vi "StringWizard.vi"() -> ()   [LabVIEW 2020]
uses:
  vi-prop-cmd.ctl
  <vilib>/Utility/miscctls.llb/LVRowAndColumnUnsignedTypeDef.ctl
  <vilib>/ErrorRing/Error Ring.xnode
panel:
  in  "reload":bool
  in  "Directory":path
  in  "Multicolumn Listbox":i32(listbox)
  in  "open":bool
  out "Icon":picture
  in  "Custom":bool
  in  "Description":string
  in  "Title":string
  out "VI Name":string
  in  "control strings":i32(listbox)
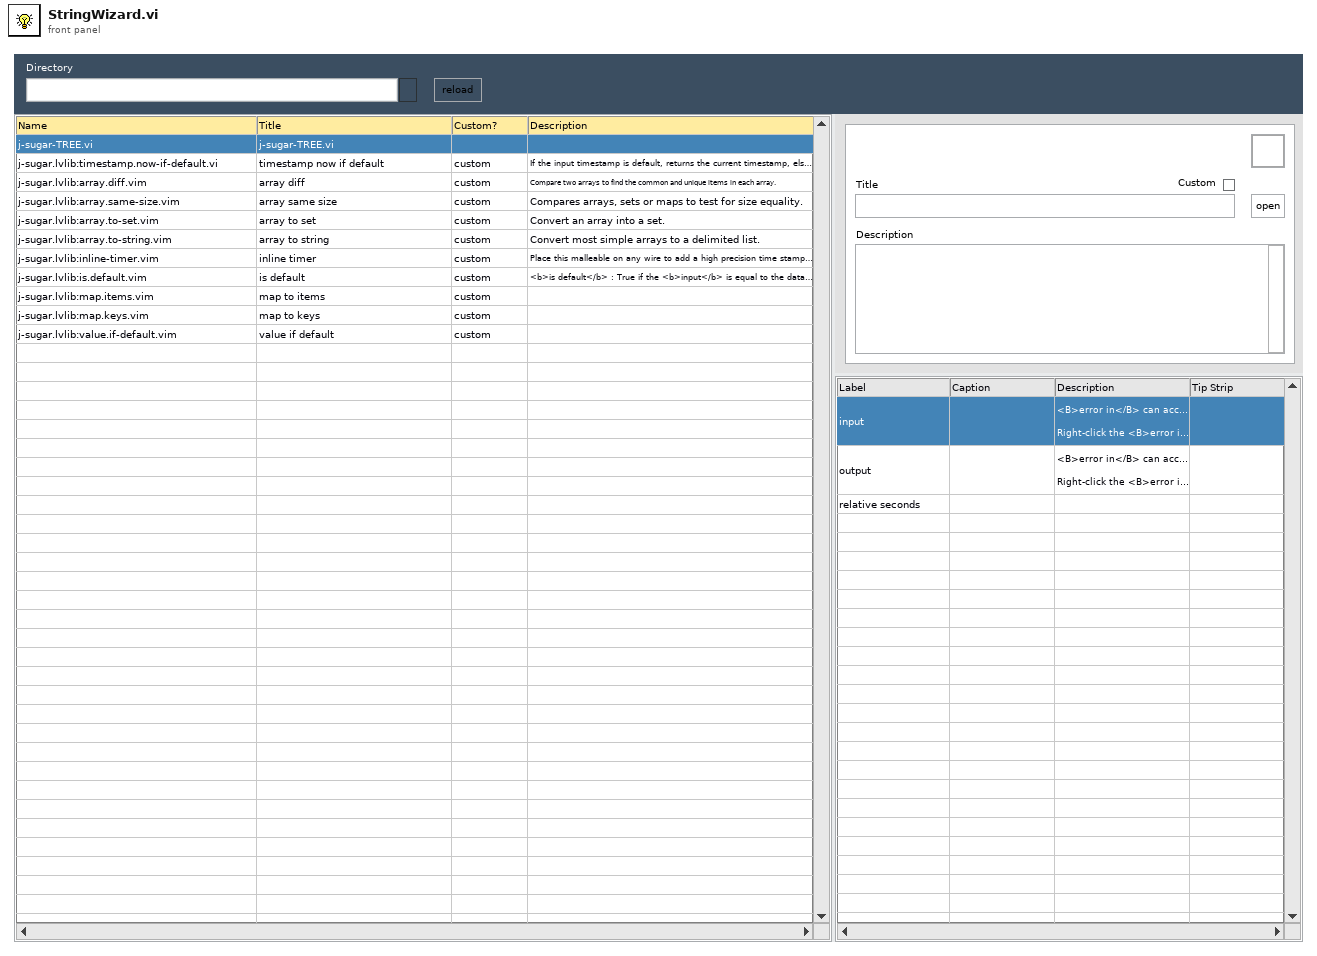
[diagram p1: front panel]
types:
  T1 = enum32{"Invalid", "Standard", "Closed", "Hidden", "Minimized", "Maximized"}
  T2 = enum32{"invalid app kind", "Development System", "Run Time System", "Student Edition", "Embedded LabVIEW", "Evaluation", "Custom"}
  T3 = typedef "LVRowAndColumnUnsignedTypeDef.ctl" = cluster{"Row":u32, "Column":u32}
  T4 = typedef "vi-prop-cmd.ctl" = cluster{"vi path":path, "property":string, "val":variant}
  T5 = cluster{"Core":cluster{"Current VI Reference":refnum<vi>, "Close Panel on Exit?":bool}, "mclb":refnum<vi>, "payload":T4, "Directory":path, "selected VI":path}
  T6 = typedef "LVRowAndColumnTypeDef.ctl" = cluster{"Row":i32, "Column":i32}
  T7 = cluster{"Current VI Reference":refnum<vi>, "Close Panel on Exit?":bool}
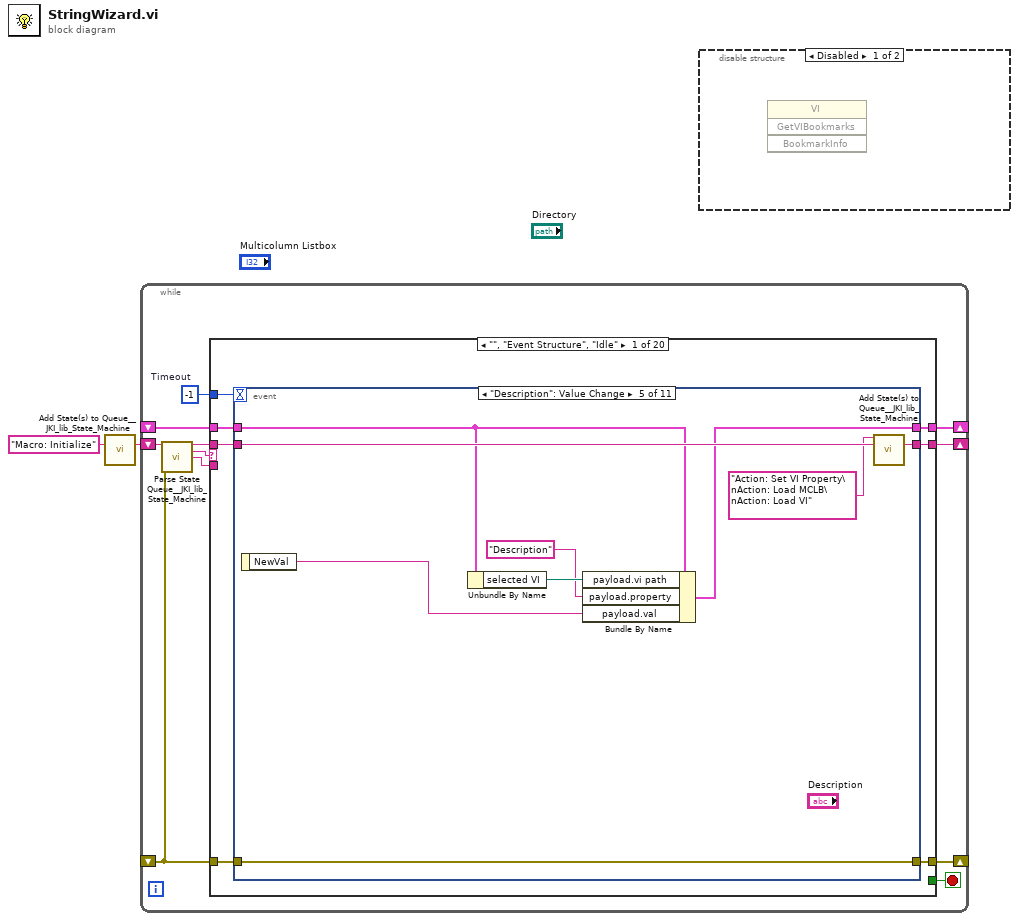
[diagram p0: block diagram]
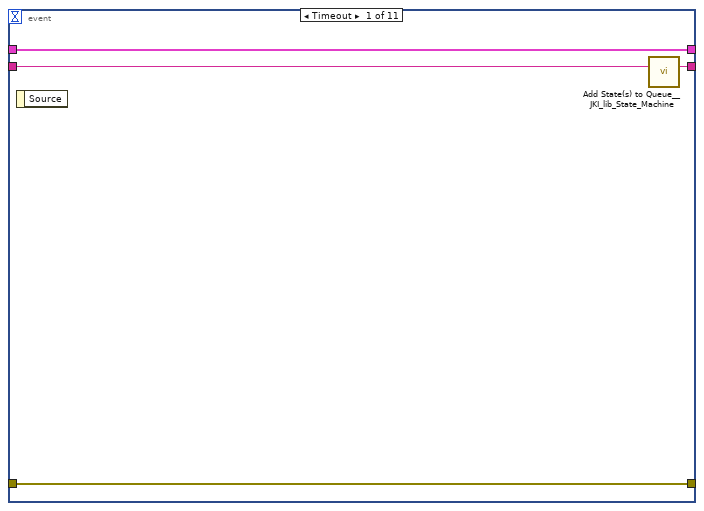
[diagram p3: hidden frame]
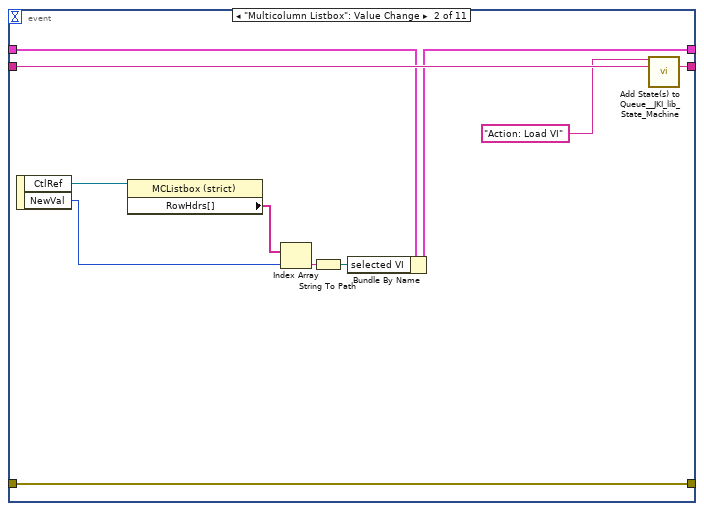
[diagram p4: hidden frame]
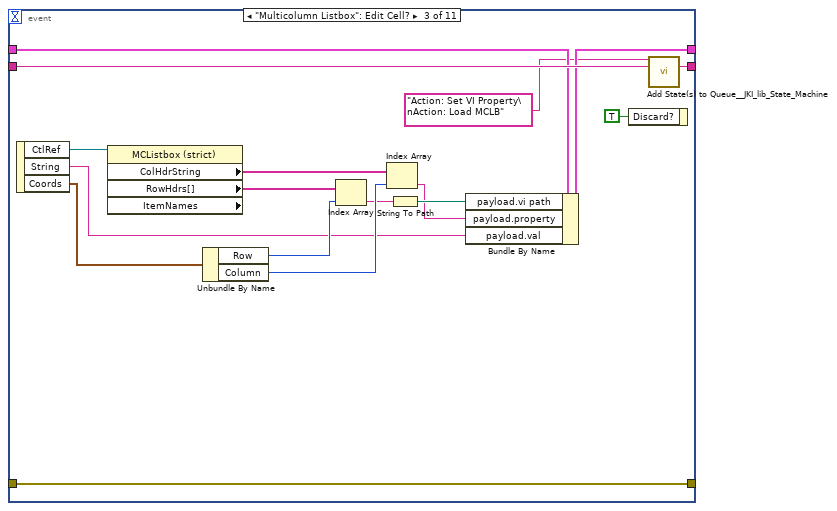
[diagram p5: hidden frame]
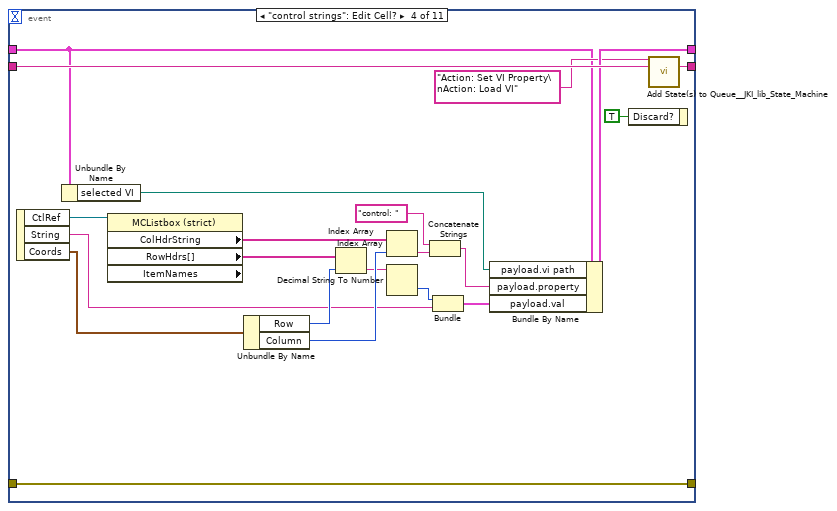
[diagram p6: hidden frame]
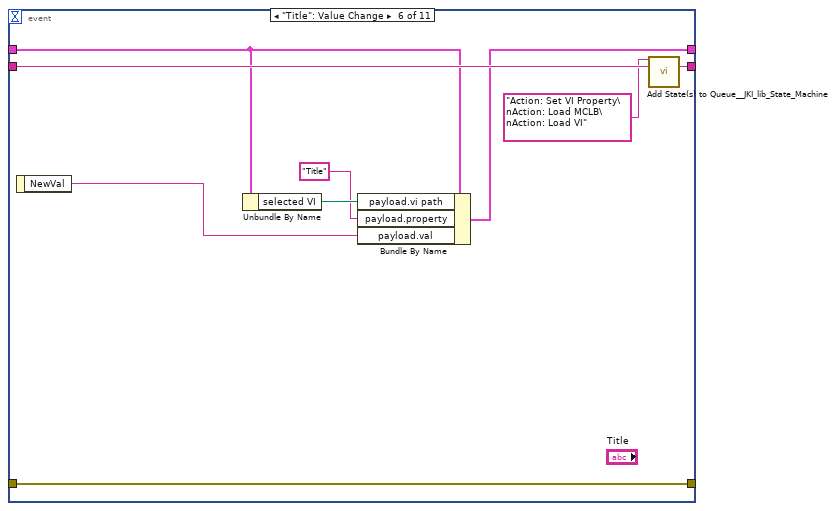
[diagram p7: hidden frame]
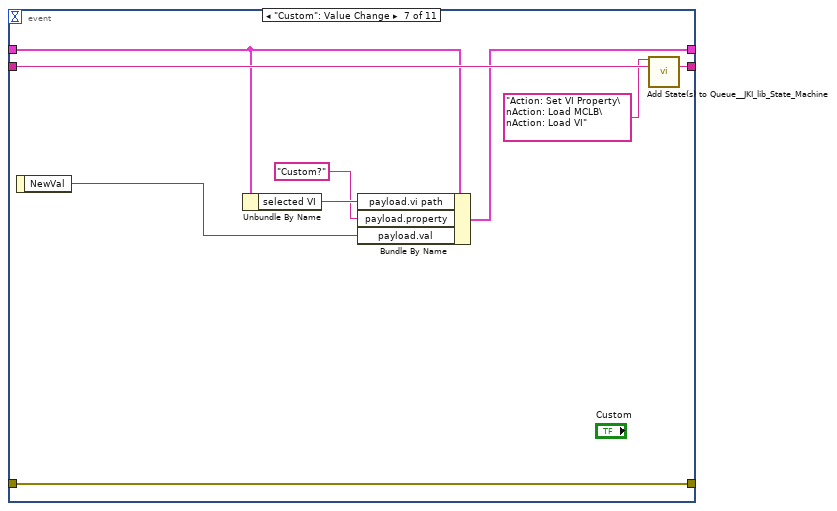
[diagram p8: hidden frame]
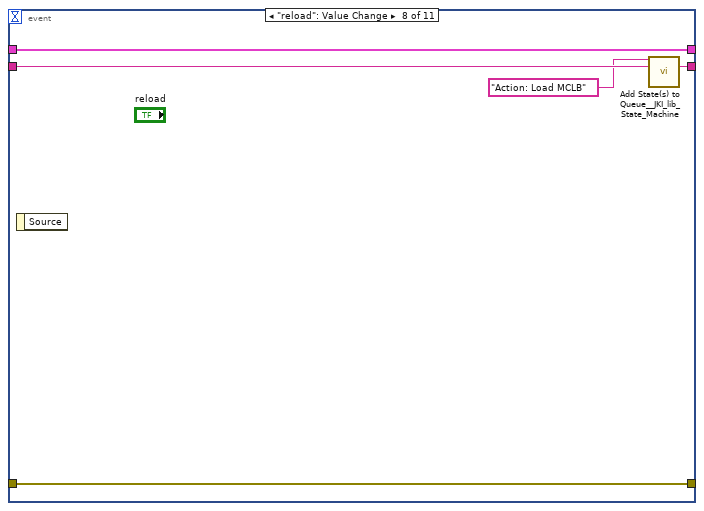
[diagram p9: hidden frame]
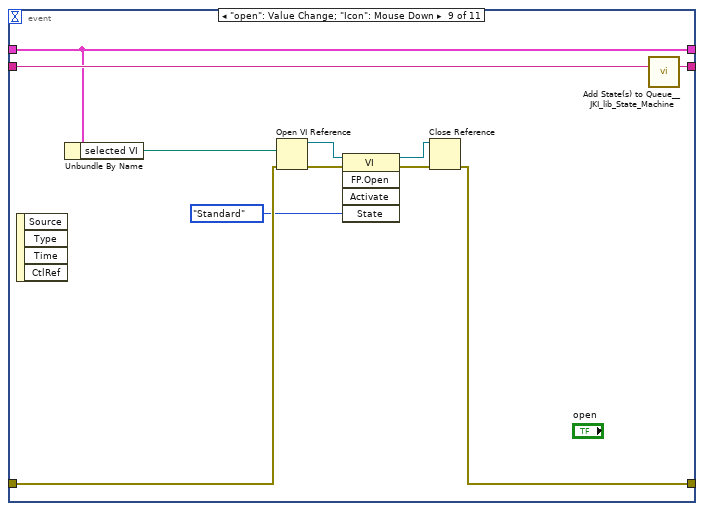
[diagram p10: hidden frame]
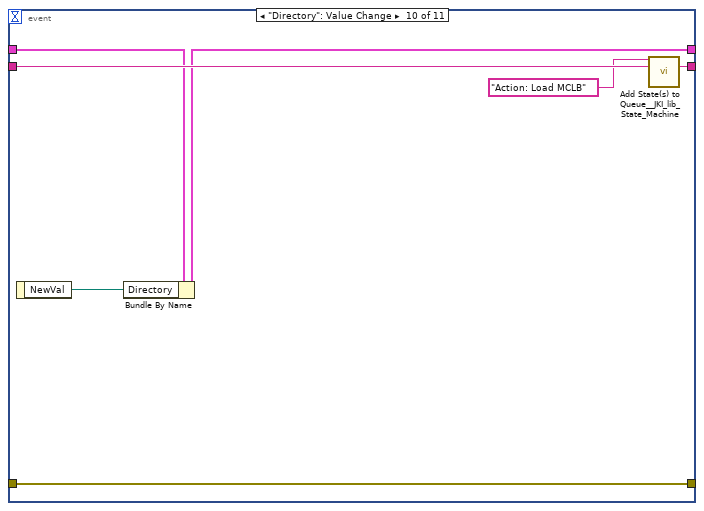
[diagram p11: hidden frame]
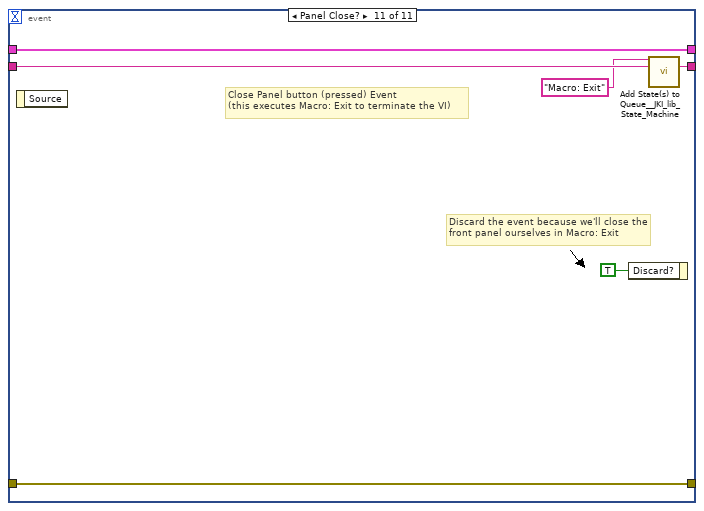
[diagram p12: hidden frame]
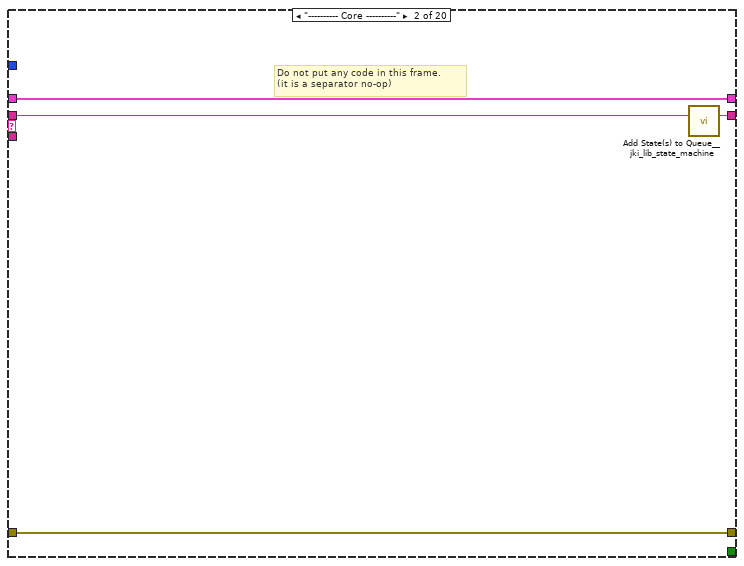
[diagram p13: hidden frame]
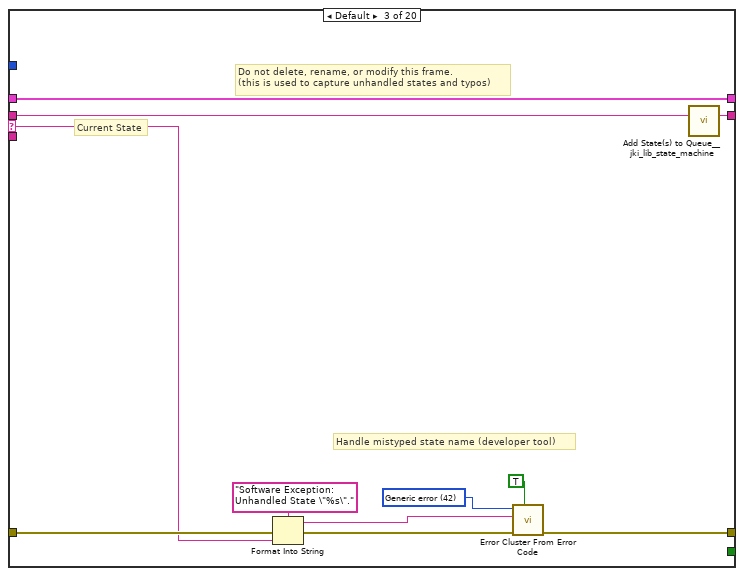
[diagram p14: hidden frame]
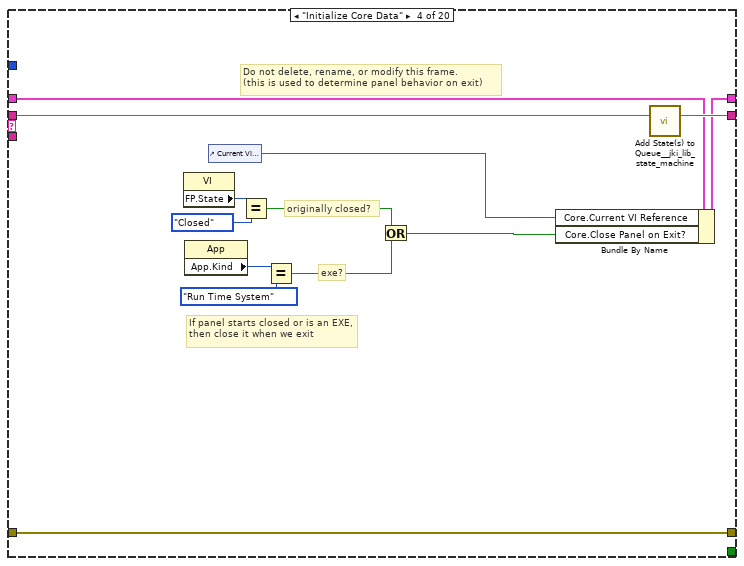
[diagram p15: hidden frame]
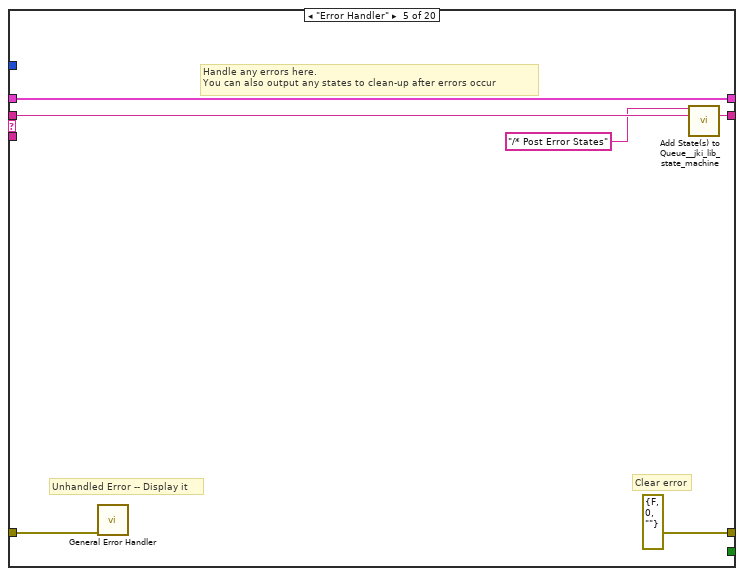
[diagram p16: hidden frame]
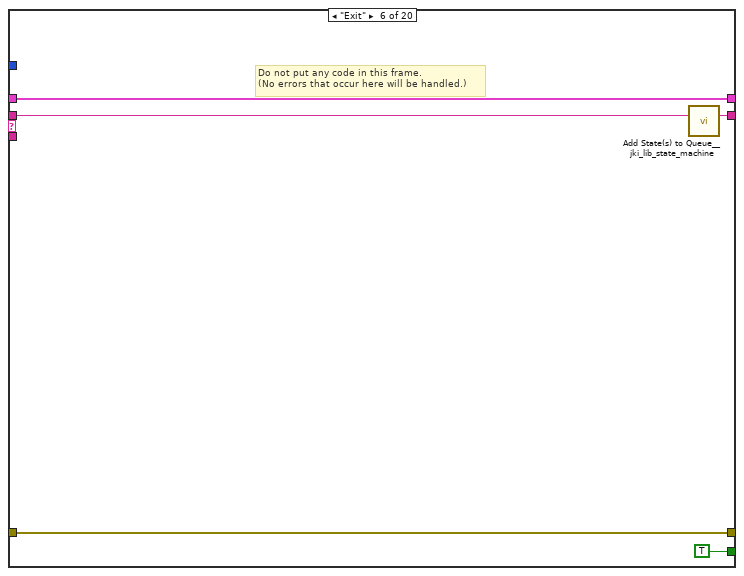
[diagram p17: hidden frame]
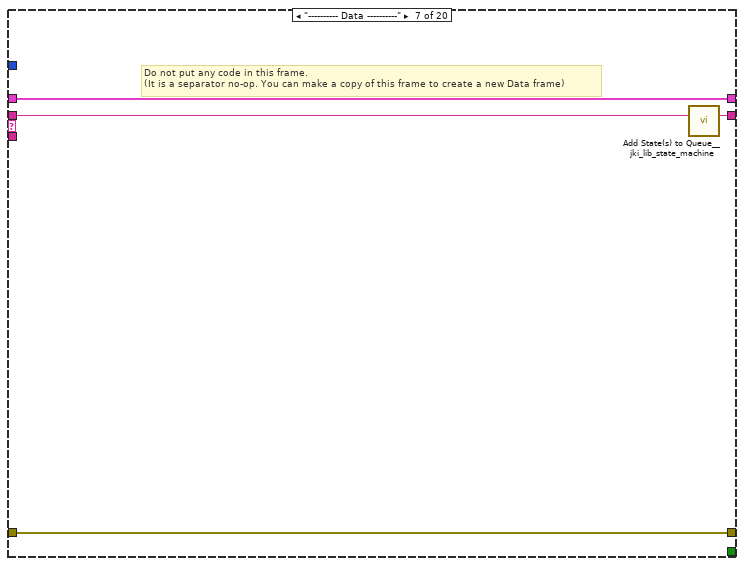
[diagram p18: hidden frame]
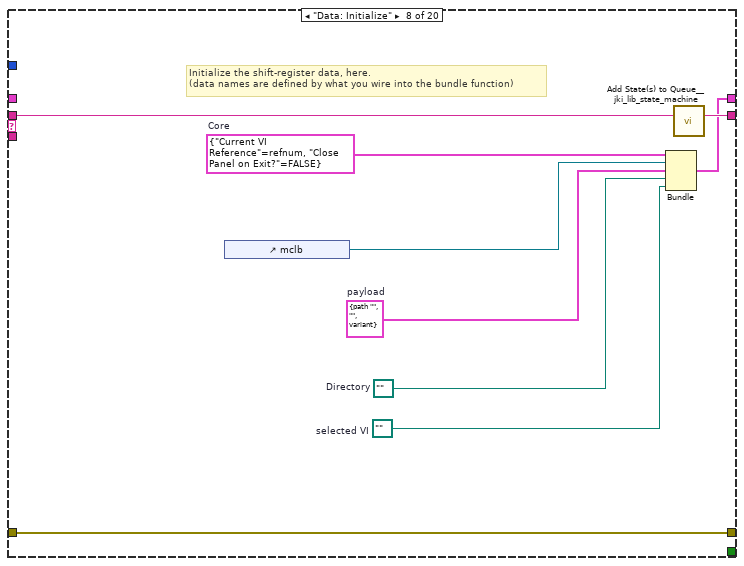
[diagram p19: hidden frame]
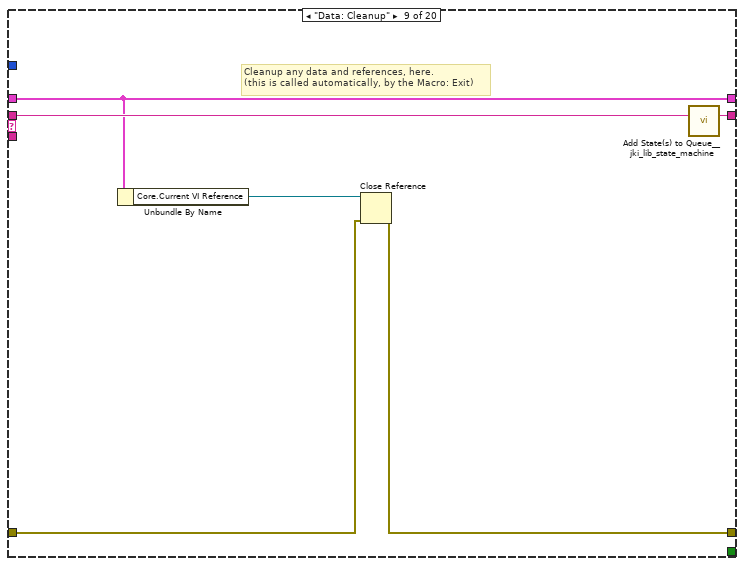
[diagram p20: hidden frame]
diagram:
  n1 = call <vilib>:"Add State(s) to Queue__JKI_lib_State_Machine.vi"("State(s) in (\"\")"="Macro: Initialize") -> ("States Out"=w2:string)  [unwired: 14 in]
  n2 = while {
    shift-right: [w6] -> _
    shift-left: _ -> [w5]
    shift-right: [w9] -> _
    shift-left: _ -> [w3]
    shift-right: [w8] -> _
    shift-left: w2 -> [w10]
    stop <- w7 stop-if-true
    w4 = -1  # Timeout
    n3 = call <vilib>:"Parse State Queue__JKI_lib_State_Machine.vi"("State Queue"=w10, "Error In (no error)"=w3) -> ("Remaining States"=w12:string, "Current State"=w13:string, "Arguments"=w11:string)  [unwired: 11 in]
    n4 = case shown="\"\", \"Event Structure\", \"Idle\"" w13 {
      selector: w13 -> [_ _ w134 _ _ _ _ _ _ _ _ _ _ _ _ _ _ _ _ _]
      tunnel: w12 -> [w20 w133 w138 w157 w163 w168 w172 w181 w187 w191 w203 w211 w222 w291 w296 w306 w310 w333 w350 w420]
      tunnel: w11 -> [_ _ _ _ _ _ _ _ _ _ _ w206 w216 _ _ _ _ _ _ _]
      tunnel: w5 -> [w18 w130 w136 w150 w160 w166 w169 _ w183 w188 w201 w209 w218 w288 w293 w303 w307 w331 w337 w413]
      tunnel: [w17 w131 w140 w154 errorcluster {"status"=FALSE, "code"=0, "source"=""} ("error out") w165 w170 w175 w184 w189 w200 w207 w219 w289 w294 w304 w308 w323 w335 w410] -> w9
      tunnel: w3 -> [w16 w131 w139 w154 w159 w165 w170 w175 w182 w189 w200 w208 w220 w289 w294 w304 w308 w330 w334 w411]
      tunnel: [w19 w132 w137 w156 w162 w167 w171 w180 w186 w190 w202 w210 w221 w290 w295 w305 w309 w332 w349 w419] -> w8
      tunnel: [_ _ _ _ _ TRUE _ _ _ _ _ _ _ _ _ _ _ _ _ _] -> w7
      tunnel: [w15 w130 w136 w155 w160 w166 w169 w179 w183 w188 w201 w209 w218 w288 w293 w303 w307 w331 w338 w413] -> w6
      tunnel: w4 -> [w14 _ _ _ _ _ _ _ _ _ _ _ _ _ _ _ _ _ _ _]
      frame "", "Event Structure", "Idle" {
        n5 = event shown="[4] \"Description\": Value Change" {
          selector: _ -> [_ _ _ _ _ _ _ _ _ _ _]
          dyn-events: _ -> [_ _ _ _ _ _ _ _ _ _ _]
          timeout: w14 -> [_ _ _ _ _ _ _ _ _ _ _]
          tunnel: w20 -> [w24 w35 w52 w73 w82 w91 w100 w105 w116 w123 w129]
          tunnel: [w23 w34 w51 w72 w81 w90 w99 w104 w115 w122 w128] -> w19
          tunnel: w18 -> [w21 w32 w44 w61 w77 w86 w95 w102 w114 w117 w126]
          tunnel: [w22 w33 w50 w71 w80 w89 w98 w103 w109 w121 w127] -> w17
          tunnel: w16 -> [w22 w33 w50 w71 w80 w89 w98 w103 w108 w121 w127]
          tunnel: [w21 w26 w45 w66 w79 w88 w97 w102 w114 w118 w126] -> w15
          event Timeout {
            n6 = event-data() -> ()  [unwired: 1 in, 1 out]
            n7 = call <vilib>:"Add State(s) to Queue__JKI_lib_State_Machine.vi"("State(s) in (\"\")"=w24) -> ("States Out"=w23:string)  [unwired: 14 in]
          }
          event "Multicolumn Listbox": Value Change {
            n8 = event-data() -> ("CtlRef"=w31:refnum<vi>, "NewVal"=w29:i32)  [unwired: 1 in]
            n9 = property on="Property Node" class="MCListbox (strict)"(reference=w31) -> ("RowHdrs[]"=w30:string[])  [unwired: 1 in, 2 out]
            n10 = Index Array(array=w30, index=w29) -> (element=w28:string)
            n11 = String To Path(string=w28) -> (path=w25:path)
            n12 = Bundle By Name(cluster=w32, "selected VI"=w25) -> (w26:T5)
            n13 = call <vilib>:"Add State(s) to Queue__JKI_lib_State_Machine.vi"("State(s) in Front (\"\")"="Action: Load VI", "State(s) in (\"\")"=w35) -> ("States Out"=w34:string)  [unwired: 13 in]
          }
          event "Multicolumn Listbox": Edit Cell? {
            n14 = event-data() -> ("CtlRef"=w47:refnum<vi>, "String"=w38:string, "Coords"=w36:T6)  [unwired: 1 in]
            n15 = property on="Property Node" class="MCListbox (strict)" props=["ColHdrString", "RowHdrs[]", "ItemNames"](reference=w47) -> ("ColHdrString"=w49:string[], "RowHdrs[]"=w48:string[])  [unwired: 1 in, 3 out]
            n16 = Unbundle By Name(w36) -> ("Row"=w43:i32, "Column"=w42:i32)
            n17 = Index Array(array=w48, index=w43) -> (element=w41:string)
            n18 = Index Array(array=w49, index=w42) -> (element=w39:string)
            n19 = String To Path(string=w41) -> (path=w40:path)
            n20 = Bundle By Name(cluster=w44, "payload.vi path"=w40, "payload.property"=w39, "payload.val"=w38) -> (w45:T5)
            n21 = event-data("Discard?"=TRUE) -> ()  [unwired: 1 in, 1 out]
            n22 = call <vilib>:"Add State(s) to Queue__JKI_lib_State_Machine.vi"("State(s) in Front (\"\")"="Action: Set VI Property\nAction: Load MCLB", "State(s) in (\"\")"=w52) -> ("States Out"=w51:string)  [unwired: 13 in]
          }
          event "control strings": Edit Cell? {
            n23 = event-data() -> ("CtlRef"=w68:refnum<vi>, "String"=w56:string, "Coords"=w62:T6)  [unwired: 1 in]
            n24 = Unbundle By Name(w61) -> ("selected VI"=w60:path)
            n25 = property on="Property Node" class="MCListbox (strict)" props=["ColHdrString", "RowHdrs[]", "ItemNames"](reference=w68) -> ("ColHdrString"=w70:string[], "RowHdrs[]"=w69:string[])  [unwired: 1 in, 3 out]
            n26 = Unbundle By Name(w62) -> ("Row"=w65:i32, "Column"=w64:i32)
            n27 = Index Array(array=w69, index=w65) -> (element=w54:string)
            n28 = Index Array(array=w70, index=w64) -> (element=w58:string)
            n29 = Decimal String To Number(string=w54) -> (number=w53:i32)  [unwired: 2 in, 1 out]
            n30 = Concatenate Strings("control: ", w58) -> (w57:string)
            n31 = Bundle(w53, "String"=w56) -> (w55:cluster{i32, "String":string})  [unwired: 1 in]
            n32 = Bundle By Name(cluster=w61, "payload.vi path"=w60, "payload.property"=w57, "payload.val"=w55) -> (w66:T5)
            n33 = event-data("Discard?"=TRUE) -> ()  [unwired: 1 in, 1 out]
            n34 = call <vilib>:"Add State(s) to Queue__JKI_lib_State_Machine.vi"("State(s) in Front (\"\")"="Action: Set VI Property\nAction: Load VI", "State(s) in (\"\")"=w73) -> ("States Out"=w72:string)  [unwired: 13 in]
          }
          event "Description": Value Change {
            n35 = event-data() -> ("NewVal"=w76:string)  [unwired: 1 in]
            n36 = Unbundle By Name(w77) -> ("selected VI"=w75:path)
            n37 = Bundle By Name(cluster=w77, "payload.vi path"=w75, "payload.property"="Description", "payload.val"=w76) -> (w79:T5)
            n38 = call <vilib>:"Add State(s) to Queue__JKI_lib_State_Machine.vi"("State(s) in Front (\"\")"="Action: Set VI Property\nAction: Load MCLB\nAction: Load VI", "State(s) in (\"\")"=w82) -> ("States Out"=w81:string)  [unwired: 13 in]
          }
          event "Title": Value Change {
            n39 = event-data() -> ("NewVal"=w85:string)  [unwired: 1 in]
            n40 = Unbundle By Name(w86) -> ("selected VI"=w84:path)
            n41 = Bundle By Name(cluster=w86, "payload.vi path"=w84, "payload.property"="Title", "payload.val"=w85) -> (w88:T5)
            n42 = call <vilib>:"Add State(s) to Queue__JKI_lib_State_Machine.vi"("State(s) in Front (\"\")"="Action: Set VI Property\nAction: Load MCLB\nAction: Load VI", "State(s) in (\"\")"=w91) -> ("States Out"=w90:string)  [unwired: 13 in]
          }
          event "Custom": Value Change {
            n43 = event-data() -> ("NewVal"=w94:bool)  [unwired: 1 in]
            n44 = Unbundle By Name(w95) -> ("selected VI"=w93:path)
            n45 = Bundle By Name(cluster=w95, "payload.vi path"=w93, "payload.property"="Custom?", "payload.val"=w94) -> (w97:T5)
            n46 = call <vilib>:"Add State(s) to Queue__JKI_lib_State_Machine.vi"("State(s) in Front (\"\")"="Action: Set VI Property\nAction: Load MCLB\nAction: Load VI", "State(s) in (\"\")"=w100) -> ("States Out"=w99:string)  [unwired: 13 in]
          }
          event "reload": Value Change {
            n47 = event-data() -> ()  [unwired: 1 in, 1 out]
            n48 = call <vilib>:"Add State(s) to Queue__JKI_lib_State_Machine.vi"("State(s) in Front (\"\")"="Action: Load MCLB", "State(s) in (\"\")"=w105) -> ("States Out"=w104:string)  [unwired: 13 in]
          }
          event "open": Value Change; "Icon": Mouse Down {
            n49 = event-data() -> ()  [unwired: 1 in, 4 out]
            n50 = Unbundle By Name(w114) -> ("selected VI"=w113:path)
            n51 = Open VI Reference(vi path=w113, error in (no error)=w108) -> (vi reference=w106:refnum<vi>, error out=w112:errorcluster)  [unwired: 4 in]
            n52 = invoke class="VI" method="FP.Open"(reference=w106, error in=w112, "State"=T1."Standard") -> (reference out=w110:refnum<vi>, error out=w111:errorcluster)  [unwired: 2 in, 3 out]
            n53 = Close Reference(reference=w110, error in (no error)=w111) -> (error out=w109:errorcluster)
            n54 = call <vilib>:"Add State(s) to Queue__JKI_lib_State_Machine.vi"("State(s) in (\"\")"=w116) -> ("States Out"=w115:string)  [unwired: 14 in]
          }
          event "Directory": Value Change {
            n55 = event-data() -> ("NewVal"=w119:path)  [unwired: 1 in]
            n56 = Bundle By Name(cluster=w117, "Directory"=w119) -> (w118:T5)
            n57 = call <vilib>:"Add State(s) to Queue__JKI_lib_State_Machine.vi"("State(s) in Front (\"\")"="Action: Load MCLB", "State(s) in (\"\")"=w123) -> ("States Out"=w122:string)  [unwired: 13 in]
          }
          event Panel Close? {
            # "Discard the event because we'll close the front panel ourselves in Macro: Exit"
            # "Close Panel button (pressed) Event\n(this executes Macro: Exit to terminate the VI)"
            n58 = event-data() -> ()  [unwired: 1 in, 1 out]
            n59 = event-data("Discard?"=TRUE) -> ()  [unwired: 1 in, 1 out]
            n60 = call <vilib>:"Add State(s) to Queue__JKI_lib_State_Machine.vi"("State(s) in Front (\"\")"="Macro: Exit", "State(s) in (\"\")"=w129) -> ("States Out"=w128:string)  [unwired: 13 in]
          }
        }
      }
      frame "---------- Core ----------" {
        # "Do not put any code in this frame.\n(it is a separator no-op)"
        n61 = call <vilib>:"Add State(s) to Queue__jki_lib_state_machine.vi"("State(s) in (\"\")"=w133) -> ("States Out"=w132:string)  [unwired: 14 in]
      }
      frame Default {
        w143 = 42 items=["No error", "Argument error", "Memory is full", "Out of zone", "End of file", "File already open", "Generic file I/O error", "File not found", "File permission error", "Disk is full", "Duplicate path", "Too many files open", "System feature not enabled", "Resource file not found", "Cannot add resource", "Resource not found", "Image not found", "Image memory error", "Pen does not exist", "Config type invalid", "Config token not found", "Config parse error", "Config memory error", "Bad external code format", "Bad external code offset", "External code not present", "Null window", "Destroy window error", "Null menu", "Print aborted", "Bad print record", "Print driver error", "Windows error during printing", "Memory error during printing", "Print dialog error", "Generic print error", "Invalid device refnum", "Device not found", "Device parameter error", "Device unit error", "Cannot open device", "Device call aborted", "Generic error", "Cancelled by user", "Object ID too low", "Object ID too high", "Object not in heap", "Unknown heap", "Unknown object (invalid DefProc)", "Unknown object (DefProc not in table)", "Message out of range", "Invalid (null) method", "Unknown message", "Manager call not supported", "Bad address", "Network operation in progress", "Network operation timed out", "Connection is busy", "Network attribute not supported", "Network error", "Address in use", "System out of memory", "Connection aborted", "Connection refused", "Not connected", "Already connected", "Connection closed", "Initialization error (interapplication manager)", "Bad occurrence", "Wait on unbound occurrence handler", "Occurrence queue overflow", "Datalog type conflict", "Unused", "Unrecognized type (interapplication manager)", "Memory corrupt", "Failed to make temporary DLL", "Old CIN version", "Drag socket not found", "Failed to load drop-object", "Failed to register OLE object", "Failed to release OLE object", "Format specifier type mismatch", "Unknown format specifier", "Too few format specifiers", "Too many format specifiers", "Scan failed", "Newer CIN version", "Error converting to variant", "Runtime menu error", "Password tampered", "Variant attribute not found", "Incompatible variant data type", "Event data is not available", "Event Store is not present", "Occurrence is not found", "Event Queue is not created", "Event info is not available", "Refnum passed is NULL", "Error retrieving Class GUID", "Error retrieving CoClass GUID", "Error retrieving TypeLib GUID.", "Bad built application magic bytes.", "Specific driver is different from the specific driver associated with the Logical Name.", "There is no session opened to the class driver.", "Max Error", "MAX - Error with config objects", "MAX - Error loading configuration", "MAX - Group not supported"]
        # "Current State"
        # "Do not delete, rename, or modify this frame.\n(this is used to capture unhandled states and typos)"
        # "Handle mistyped state name (developer tool)"
        n62 = Format Into String(format string="Software Exception: Unhandled State \"%s\"." ("message"), error in=w139, w134) -> (resulting string=w142:string, error out=w141:errorcluster)  [unwired: 1 in]
        n63 = call <vilib>:"Error Cluster From Error Code.vi"("show call chain? (False)"=TRUE, "error in (no error)"=w141, "error message (\"\")"=w142, "error code (0)"=w143) -> ("error out"=w140:errorcluster)  [unwired: 5 in]
        n64 = call <vilib>:"Add State(s) to Queue__jki_lib_state_machine.vi"("State(s) in (\"\")"=w138) -> ("States Out"=w137:string)  [unwired: 14 in]
      }
      frame "Initialize Core Data" {
        # "Do not delete, rename, or modify this frame.\n(this is used to determine panel behavior on exit)"
        # "originally closed?"
        # "exe?"
        # "If panel starts closed or is an EXE, then close it when we exit"
        n65 = property class="VI"() -> ("FP.State"=w147:T1)  [unwired: 2 in, 2 out]
        n66 = property class="App"() -> ("App.Kind"=w153:T2)  [unwired: 2 in, 2 out]
        n67 = control-ref of="Current VI Reference"() -> (w148:refnum<vi>)
        n68 = Equal?(x=w147, y=T1."Closed" ("Front Panel Window:State")) -> (x = y?=w145:bool)
        n69 = Equal?(x=w153, y=T2."Run Time System" ("Application:Kind")) -> (x = y?=w151:bool)
        n70 = Or(x=w145, y=w151) -> (x .or. y?=w149:bool)
        n71 = Bundle By Name(cluster=w150, "Core.Current VI Reference"=w148, "Core.Close Panel on Exit?"=w149) -> (w155:T5)
        n72 = call <vilib>:"Add State(s) to Queue__jki_lib_state_machine.vi"("State(s) in (\"\")"=w157) -> ("States Out"=w156:string)  [unwired: 14 in]
      }
      frame "Error Handler" {
        # "Unhandled Error -- Display it"
        # "Handle any errors here.\nYou can also output any states to clean-up after errors occur"
        # "Clear error"
        n73 = call <vilib>:"General Error Handler.vi"("error in (no error)"=w159) -> ()  [unwired: 10 in, 5 out]
        n74 = call <vilib>:"Add State(s) to Queue__jki_lib_state_machine.vi"("State(s) in Front (\"\")"="/* Post Error States", "State(s) in (\"\")"=w163) -> ("States Out"=w162:string)  [unwired: 13 in]
      }
      frame "Exit" {
        # "Do not put any code in this frame.\n(No errors that occur here will be handled.)"
        n75 = call <vilib>:"Add State(s) to Queue__jki_lib_state_machine.vi"("State(s) in (\"\")"=w168) -> ("States Out"=w167:string)  [unwired: 14 in]
      }
      frame "---------- Data ----------" {
        # "Do not put any code in this frame.\n(It is a separator no-op. You can make a copy of this frame to create a new Data frame)"
        n76 = call <vilib>:"Add State(s) to Queue__jki_lib_state_machine.vi"("State(s) in (\"\")"=w172) -> ("States Out"=w171:string)  [unwired: 14 in]
      }
      frame "Data: Initialize" {
        w173 = path ""  # selected VI
        w174 = path ""  # Directory
        w176 = T4 {"vi path"=path "", "property"="", "val"=variant}  # payload
        w178 = T7 {"Current VI Reference"=refnum, "Close Panel on Exit?"=FALSE}  # Core
        # "Initialize the shift-register data, here.\n(data names are defined by what you wire into the bundle function)"
        n77 = control-ref of="mclb"() -> (w177:refnum<vi>)
        n78 = Bundle("Core"=w178, "mclb"=w177, "payload"=w176, "Directory"=w174, "selected VI"=w173) -> (w179:T5)  [unwired: 1 in]
        n79 = call <vilib>:"Add State(s) to Queue__jki_lib_state_machine.vi"("State(s) in (\"\")"=w181) -> ("States Out"=w180:string)  [unwired: 14 in]
      }
      frame "Data: Cleanup" {
        # "Cleanup any data and references, here.\n(this is called automatically, by the Macro: Exit)"
        n80 = Unbundle By Name(w183) -> ("Core.Current VI Reference"=w185:refnum<vi>)
        n81 = Close Reference(reference=w185, error in (no error)=w182) -> (error out=w184:errorcluster)
        n82 = call <vilib>:"Add State(s) to Queue__jki_lib_state_machine.vi"("State(s) in (\"\")"=w187) -> ("States Out"=w186:string)  [unwired: 14 in]
      }
      frame "---------- UI ----------" {
        # "Do not put any code in this frame.\n(It is a separator no-op. You can make a copy of this frame to create a new UI frame)"
        n83 = call <vilib>:"Add State(s) to Queue__jki_lib_state_machine.vi"("State(s) in (\"\")"=w191) -> ("States Out"=w190:string)  [unwired: 14 in]
      }
      frame "UI: Initialize" {
        w195 = ""
        w192 = string[][] [] ("Item Names")
        w199 = string[] [] ("Column Header Strings[]")
        # "Pre-load the path if its already loaded"
        # "Initialize the User Interface, here.\n(this is called automatically, by the Macro: Init)"
        n84 = property on="Directory" class="Path"() -> (error out=w198:errorcluster, "Value"=w197:path)  [unwired: 2 in, 1 out]
        n85 = Empty String/Path?(string/path=w197) -> (empty?=w196:bool)
        n86 = case shown="True" w196 {
          tunnel: w197 -> [w205 _]
          tunnel: w198 -> [w204 _]
          frame False {
            n87 = property on="Directory" class="Path"(error in=w204, "Val(Sgnl)"=w205) -> ()  [unwired: 1 in, 2 out]
          }
          frame True {
            # "empty"
          }
        }
        n88 = local write "VI Name"(w195) -> ()
        n89 = local write "Title"(w195) -> ()
        n90 = local write "Description"(w195) -> ()
        n91 = local write "Custom"(FALSE ("Custom")) -> ()
        n92 = property on="Multicolumn Listbox" class="MCListbox (strict)"("ItemNames"=w192, "ColHdrString"=w199, "RowHdrs[]"=w199, "TopLeft"=T3 {"Row"=0, "Column"=0} ("Top Left Visible Cell")) -> ()  [unwired: 2 in, 2 out]
        n93 = property on="control strings" class="MCListbox (strict)"("ItemNames"=w192) -> ()  [unwired: 2 in, 2 out]
        n94 = call <vilib>:"Add State(s) to Queue__jki_lib_state_machine.vi"("State(s) in (\"\")"=w203) -> ("States Out"=w202:string)  [unwired: 14 in]
      }
      frame "UI: Cursor Set" {
        # "Argument"
        # "Set and Unset Cursor Busy.\n(Usage: \"UI: Cursor Set >> Busy|Idle\")"
        n95 = case shown="\"Idle\", Default" w206 {
          tunnel: w208 -> [w213 w215]
          tunnel: [w212 w214] -> w207
          frame "Idle", Default {
            n96 = call <vilib>:"Unset Busy.vi"("error in (no error)"=w213) -> ("error out"=w212:errorcluster)  [unwired: 10 in]
          }
          frame "Busy" {
            n97 = call <vilib>:"Set Busy.vi"("error in (no error)"=w215) -> ("error out"=w214:errorcluster)  [unwired: 9 in, 1 out]
          }
        }
        n98 = call <vilib>:"Add State(s) to Queue__jki_lib_state_machine.vi"("State(s) in (\"\")"=w211) -> ("States Out"=w210:string)  [unwired: 14 in]
      }
      frame "UI: Front Panel State" {
        # "Argument"
        # "Set Front Panel Open or Closed\n(Usage: \"UI: Front Panel State >> Open|Close\")"
        n99 = Unbundle By Name(w218) -> ("Core.Current VI Reference"=w217:refnum<vi>)
        n100 = case shown="\"Minimize\", \"Minimized\"" w216 {
          tunnel: w220 -> [w228 w243 w254 w267 w280]
          tunnel: [w230 w244 w256 w269 w282] -> w219
          tunnel: w217 -> [w229 w241 w255 w268 w281]
          frame "Open", "Standard", Default {
            w223 = T1."Standard" ("State")
            n101 = property class="VI"(reference=w229, error in=w228) -> (reference out=w226:refnum<vi>, error out=w227:errorcluster, "FP.State"=w225:T1)
            n102 = Not Equal?(x=w225, y=w223) -> (x != y?=w224:bool)
            n103 = case shown="True" w224 {
              tunnel: [w234 w236] -> w230
              tunnel: w227 -> [w233 w236]
              tunnel: w226 -> [w232 _]
              tunnel: w223 -> [w231 _]
              frame True {
                n104 = invoke class="VI" method="FP.Open"(reference=w232, error in=w233, "Activate"=TRUE, "State"=w231) -> (error out=w234:errorcluster)  [unwired: 1 in, 4 out]
              }
              frame False {
              }
            }
          }
          frame "Close", "Closed" {
            n105 = property class="VI"(reference=w241, error in=w243) -> (reference out=w240:refnum<vi>, error out=w242:errorcluster, "FP.State"=w238:T1)
            n106 = Not Equal?(x=w238, y=T1."Closed" ("Front Panel Window:State")) -> (x != y?=w237:bool)
            n107 = case shown="True" w237 {
              tunnel: [w245 w248] -> w244
              tunnel: w242 -> [w245 w247]
              tunnel: w240 -> [_ w246]
              frame False {
              }
              frame True {
                n108 = invoke class="VI" method="FP.Close"(reference=w246, error in=w247) -> (error out=w248:errorcluster)  [unwired: 1 in, 2 out]
              }
            }
          }
          frame "Hidden", "Hide" {
            w249 = T1."Hidden" ("State")
            n109 = property class="VI"(reference=w255, error in=w254) -> (reference out=w252:refnum<vi>, error out=w253:errorcluster, "FP.State"=w251:T1)
            n110 = Not Equal?(x=w251, y=w249) -> (x != y?=w250:bool)
            n111 = case shown="True" w250 {
              tunnel: [w260 w261] -> w256
              tunnel: w253 -> [w259 w261]
              tunnel: w252 -> [w258 _]
              tunnel: w249 -> [w257 _]
              frame True {
                n112 = invoke class="VI" method="FP.Open"(reference=w258, error in=w259, "State"=w257) -> (error out=w260:errorcluster)  [unwired: 2 in, 4 out]
              }
              frame False {
              }
            }
          }
          frame "Minimize", "Minimized" {
            w262 = T1."Minimized" ("State")
            n113 = property class="VI"(reference=w268, error in=w267) -> (reference out=w265:refnum<vi>, error out=w266:errorcluster, "FP.State"=w264:T1)
            n114 = Not Equal?(x=w264, y=w262) -> (x != y?=w263:bool)
            n115 = case shown="True" w263 {
              tunnel: [w273 w274] -> w269
              tunnel: w266 -> [w272 w274]
              tunnel: w265 -> [w271 _]
              tunnel: w262 -> [w270 _]
              frame True {
                n116 = invoke class="VI" method="FP.Open"(reference=w271, error in=w272, "State"=w270) -> (error out=w273:errorcluster)  [unwired: 2 in, 4 out]
              }
              frame False {
              }
            }
          }
          frame "Maximize", "Maximized" {
            w275 = T1."Maximized" ("State")
            n117 = property class="VI"(reference=w281, error in=w280) -> (reference out=w278:refnum<vi>, error out=w279:errorcluster, "FP.State"=w277:T1)
            n118 = Not Equal?(x=w277, y=w275) -> (x != y?=w276:bool)
            n119 = case shown="True" w276 {
              tunnel: [w286 w287] -> w282
              tunnel: w279 -> [w285 w287]
              tunnel: w278 -> [w284 _]
              tunnel: w275 -> [w283 _]
              frame True {
                n120 = invoke class="VI" method="FP.Open"(reference=w284, error in=w285, "State"=w283) -> (error out=w286:errorcluster)  [unwired: 2 in, 4 out]
              }
              frame False {
              }
            }
          }
        }
        n121 = call <vilib>:"Add State(s) to Queue__jki_lib_state_machine.vi"("State(s) in (\"\")"=w222) -> ("States Out"=w221:string)  [unwired: 14 in]
      }
      frame "---------- Macro ----------" {
        # "Do not put any code in this frame.\n(It is a separator no-op. You can make a copy of this frame to create a new Macro frame)"
        n122 = call <vilib>:"Add State(s) to Queue__jki_lib_state_machine.vi"("State(s) in (\"\")"=w291) -> ("States Out"=w290:string)  [unwired: 14 in]
      }
      frame "Macro: Initialize" {
        w292 = "Data: Initialize\nInitialize Core Data\nUI: Initialize\nUI: Front Panel State >> Open"  # Data: Initialize Initialize Core Data UI: Initialize UI: Front Panel State >> Open
        # "Initialization Macro\n(This is called once, when the VI starts)"
        n123 = call <vilib>:"Add State(s) to Queue__jki_lib_state_machine.vi"("State(s) in Front (\"\")"=w292, "State(s) in (\"\")"=w296) -> ("States Out"=w295:string)  [unwired: 13 in]
      }
      frame "Macro: Exit" {
        # "Exit Macro\n(This is called once, when the VI exits)"
        n124 = Unbundle By Name(w303) -> ("Core.Close Panel on Exit?"=w302:bool)
        n125 = Select(t="UI: Front Panel State >> Close", s=w302, f="") -> (s? t:f=w299:string)
        n126 = call <vilib>:"Add State(s) to Queue__jki_lib_state_machine.vi"("State(s) in (\"\")"=w299, "State(s) at Back (\"\")"="Data: Cleanup\nExit") -> ("States Out"=w297:string)  [unwired: 13 in]
        n127 = call <vilib>:"Add State(s) to Queue__jki_lib_state_machine.vi"("State(s) in Front (\"\")"=w297, "State(s) in (\"\")"=w306) -> ("States Out"=w305:string)  [unwired: 13 in]
      }
      frame "---------- Action ----------" {
        # "Template Separator\n(You can make a copy of, or modify, this frame)"
        n128 = call <vilib>:"Add State(s) to Queue__jki_lib_state_machine.vi"("State(s) in (\"\")"=w310) -> ("States Out"=w309:string)  [unwired: 14 in]
      }
      frame "Action: Load VI" {
        n129 = Unbundle By Name(w331) -> ("selected VI"=w313:path)
        n130 = Open VI Reference(vi path=w313, error in (no error)=w330) -> (vi reference=w324:refnum<vi>, error out=w317:errorcluster)  [unwired: 4 in]
        n131 = property class="VI"(reference=w324, error in=w317) -> (reference out=w322:refnum<vi>, error out=w326:errorcluster, "Name"=→"VI Name":string, "Front Panel.Title"=w325:string, "Front Panel.CustomTitle"=w316:bool, "Description"=w315:string)
        n132 = local write "Title"(w325) -> ()
        n133 = local write "Custom"(w316) -> ()
        n134 = local write "Description"(w315) -> ()
        n135 = call "control-table.build.vi"("error in (no error)"=w326, "vi ref"=w322) -> ("error out"=w327:errorcluster, "control table"=w329:string[][], "headers"=w328:string[], "control indicies"=w312:i32[])  [unwired: 6 in]
        n136 = Number To Decimal String(number=w312) -> (decimal integer string=w311:string[])  [unwired: 1 in]
        n137 = property on="control strings" class="MCListbox (strict)"(error in=w327, "RowHdrs[]"=w311, "ColHdrString"=w328, "ItemNames"=w329) -> (error out=w319:errorcluster)  [unwired: 1 in, 1 out]
        n138 = call "vi-icon.get.vi"("error in"=w319, "VI in"=w322) -> ("error out"=w320:errorcluster, "VI Icon"=→"Icon":picture, "VI out"=w321:refnum<vi>)  [unwired: 7 in]
        n139 = Close Reference(reference=w321, error in (no error)=w320) -> (error out=w323:errorcluster)
        n140 = call <vilib>:"Add State(s) to Queue__jki_lib_state_machine.vi"("State(s) in (\"\")"=w333) -> ("States Out"=w332:string)  [unwired: 14 in]
      }
      frame "Action: Set VI Property" {
        w344 = 1  # record mods
        n141 = Unbundle By Name(w337) -> ("payload.vi path"=w345:path, "payload.property"=w348:string, "payload.val"=w339:variant)
        n142 = Open VI Reference(vi path=w345, options=w344, error in (no error)=w334) -> (vi reference=w347:refnum<vi>, error out=w346:errorcluster)  [unwired: 3 in]
        n143 = case shown="\"Custom?\"" w348 {
          selector: w348 -> [w353 _ _ _ _ _]
          tunnel: [w355 w370 w377 w384 w391 w403] -> w341
          tunnel: w347 -> [w355 w370 w377 w384 w390 w402]
          tunnel: w346 -> [w354 w368 w375 w382 w395 w407]
          tunnel: [w352 w364 w372 w380 w387 w399] -> w342
          tunnel: w339 -> [_ w369 w376 w383 w396 w408]
          frame Default {
            n144 = xnode "Error Ring"("parameter 0"=w353) -> ("error out"=w351:errorcluster)
            n145 = Merge Errors(w354, w351) -> (w352:errorcluster)
          }
          frame "Title" {
            n146 = Variant To Data(error in=w368, type="", Variant=w369) -> (data=w367:string, error out=w365:errorcluster)
            n147 = property class="VI"(reference=w370, error in=w365, "Front Panel.CustomTitle"=TRUE ("Front Panel Window:Custom Title"), "Front Panel.Title"=w367) -> (error out=w364:errorcluster)  [unwired: 1 out]
          }
          frame "Description" {
            n148 = Variant To Data(error in=w375, type="", Variant=w376) -> (data=w371:string, error out=w373:errorcluster)
            n149 = property class="VI"(reference=w377, error in=w373, "Description"=w371) -> (error out=w372:errorcluster)  [unwired: 1 out]
          }
          frame "Custom?" {
            n150 = Variant To Data(error in=w382, type=FALSE, Variant=w383) -> (data=w379:bool, error out=w381:errorcluster)
            n151 = property class="VI"(reference=w384, error in=w381, "Front Panel.CustomTitle"=w379) -> (error out=w380:errorcluster)  [unwired: 1 out]
          }
          frame "control: Description" {
            n152 = Variant To Data(error in=w395, type=cluster{"index":i32, "value":string} {"index"=0, "value"=""}, Variant=w396) -> (data=w393:cluster{"index":i32, "value":string}, error out=w392:errorcluster)
            n153 = Unbundle By Name(w393) -> ("index"=w385:i32, "value"=w386:string)
            n154 = call "control.by-index.vi"("error in (no error)"=w392, "control index"=w385, "VI in"=w390) -> ("error out"=w388:errorcluster, "Ctl Refnum"=w389:refnum<vi>, "VI out"=w391:refnum<vi>)  [unwired: 6 in]
            n155 = property class="Ctl"(reference=w389, error in=w388, "Desc"=w386) -> (error out=w387:errorcluster)  [unwired: 1 out]
          }
          frame "Control: Tip Strip" {
            n156 = Variant To Data(error in=w407, type=cluster{"index":i32, "value":string} {"index"=0, "value"=""}, Variant=w408) -> (data=w405:cluster{"index":i32, "value":string}, error out=w404:errorcluster)
            n157 = Unbundle By Name(w405) -> ("index"=w397:i32, "value"=w398:string)
            n158 = call "control.by-index.vi"("error in (no error)"=w404, "control index"=w397, "VI in"=w402) -> ("error out"=w400:errorcluster, "Ctl Refnum"=w401:refnum<vi>, "VI out"=w403:refnum<vi>)  [unwired: 6 in]
            n159 = property class="Ctl"(reference=w401, error in=w400, "TipStrip"=w398) -> (error out=w399:errorcluster)  [unwired: 1 out]
          }
        }
        n160 = invoke class="VI" method="Save.Instrument"(reference=w341, error in=w342) -> (reference out=w340:refnum<vi>, error out=w343:errorcluster)  [unwired: 4 in, 4 out]
        n161 = Bundle By Name(cluster=w337, "payload"=T4 {"vi path"=path "", "property"="", "val"=variant}) -> (w338:T5)
        n162 = Close Reference(reference=w340, error in (no error)=w343) -> (error out=w335:errorcluster)
        n163 = call <vilib>:"Add State(s) to Queue__jki_lib_state_machine.vi"("State(s) in (\"\")"=w350) -> ("States Out"=w349:string)  [unwired: 14 in]
      }
      frame "Action: Load MCLB" {
        n164 = Unbundle By Name(w413) -> ("Directory"=w412:path)
        n165 = for {
          tunnel: [w424] -> w415 mode=concatenating
          tunnel: w412 -> [w423]
          tunnel: string[] ["*.vi", "*.vim", "*.vit", "*.ctl"] ("pattern") -> [w421] mode=indexing
          shift-right: [w425] -> w416
          shift-left: w411 -> [w422]
          n166 = call <vilib>:"Recursive File List.vi"("pattern"=w421, "error in (no error)"=w422, "Folder Path"=w423) -> ("error out"=w425:errorcluster, "All Files in Dir"=w424:path[])  [unwired: 4 in, 3 out]
        }
        n167 = for {
          tunnel: w415 -> [w428] mode=indexing
          shift-right: [w430] -> w410
          shift-left: w416 -> [w441]
          tunnel: [w432] -> w417 mode=indexing
          tunnel: [w427] -> w418 mode=indexing
          n168 = Open VI Reference(vi path=w428, error in (no error)=w441) -> (vi reference=w426:refnum<vi>, error out=w440:errorcluster)  [unwired: 4 in]
          n169 = property class="VI"(reference=w426, error in=w440) -> (reference out=w429:refnum<vi>, error out=w431:errorcluster, "Name"=w439:string, "Front Panel.Title"=w438:string, "Front Panel.CustomTitle"=w436:bool, "Description"=w437:string)
          n170 = Select(t="custom", s=w436, f="") -> (s? t:f=w433:string)
          n171 = Path To String(path=w428) -> (string=w427:string)
          n172 = Close Reference(reference=w429, error in (no error)=w431) -> (error out=w430:errorcluster)
          n173 = Build Array(w439, w438, w433, w437) -> (w432:string[])
        }
        n174 = property on="Multicolumn Listbox" class="MCListbox (strict)"("ColHdrString"=string[] ["Name", "Title", "Custom?", "Description"], "RowHdrs[]"=w418, "ItemNames"=w417) -> ()  [unwired: 2 in, 2 out]
        n175 = call <vilib>:"Add State(s) to Queue__jki_lib_state_machine.vi"("State(s) in (\"\")"=w420) -> ("States Out"=w419:string)  [unwired: 14 in]
      }
    }
  }
  n176 = disable-structure shown="Disabled" {
    frame Disabled {
      n177 = invoke class="VI" method="GetVIBookmarks"() -> ()  [unwired: 4 in, 4 out]
    }
    frame Enabled {
    }
  }
